vi "Drive_Constants.vi"() -> (20 "Position accuracy (m)":dbl=0.05, 21 "Speed step (m/s)":dbl=0.005, 22 "Wheels interval (m)":dbl=0.6, 23 "Speed convert constant":dbl=0.6, 24 "Position control loop period (ms)":i64, 25 "Turning correction constant":dbl=0.05)   [LabVIEW 2009, in "Drive.lvlib" / "Drive_Utils.lvlib"]
doc: "This VI contains the parameters used in robot driving"
uses:
  Drive_Utils.lvlib
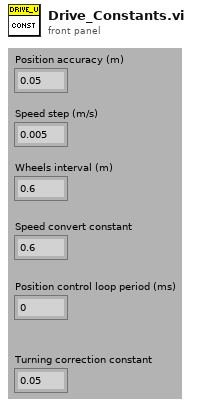
[diagram p1: front panel]
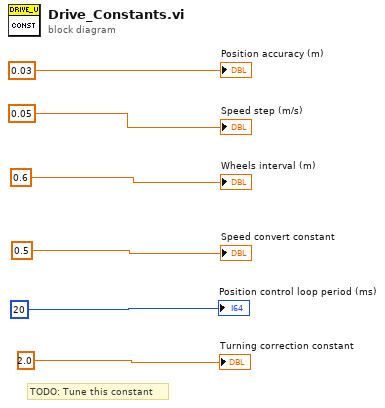
[diagram p0: block diagram]
diagram:
  # "TODO: Tune this constant"
  "Position accuracy (m)" <- 0.03 ("Position accuracy")
  "Speed step (m/s)" <- 0.05 ("Position accuracy")
  "Wheels interval (m)" <- 0.6 ("Wheels interval")
  "Speed convert constant" <- 0.5 ("Speed convert constant")
  "Position control loop period (ms)" <- i64 20 ("Position control loop period")
  "Turning correction constant" <- 2.0 ("Turning correction constance")
